vi "Average.vi"(8 "y":dbl, 11 "x":dbl) -> (1 "Average":dbl)   [LabVIEW 2013]
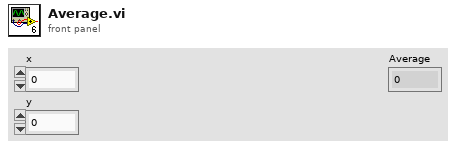
[diagram p1: front panel]
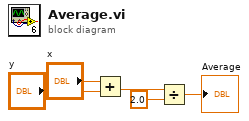
[diagram p0: block diagram]
diagram:
  n1 = Add(x="x", y="y") -> (x+y=w5:dbl)
  n2 = Divide(x=w5, y=2.0) -> (x/y=→"Average":dbl)
